vi "motorcontrol.vi"(0 "Ring":u16(ring) items=["Horizontal", "Vertical"], 1 "Direction":bool=TRUE, 2 "Frequency":dbl, 3 "# of steps":i32=1000, 4 "error in":errorcluster) -> (5 "error out":errorcluster)   [LabVIEW 2018]
uses:
  <vilib>/DAQmx/write.llb/DAQmx Write (Digital Bool 1Line 1Point).vi
  <vilib>/DAQmx/create/channels.llb/DAQmx Create Channel (DO-Digital Output).vi
  <vilib>/DAQmx/miscellaneous.llb/DAQmx Fill In Error Info.vi
  <vilib>/DAQmx/create/channels.llb/DAQmx Create Channel (CO-Pulse Generation-Frequency).vi
  <vilib>/DAQmx/configure/timing.llb/DAQmx Timing (Implicit).vi
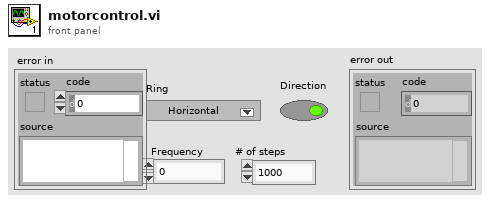
[diagram p1: front panel]
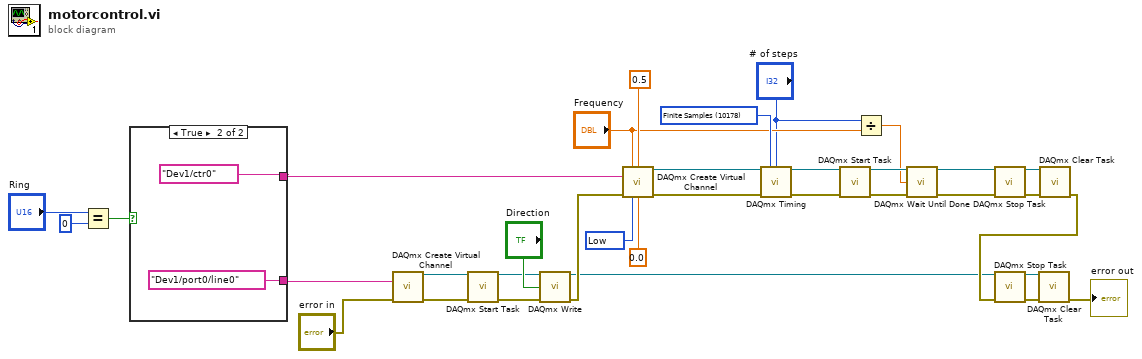
[diagram p0: block diagram]
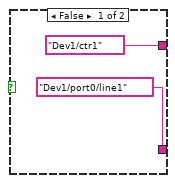
[diagram p2: hidden frame]
diagram:
  w26 = 10214 items=["High"=10192, "Low"=10214] ("idle state")
  w34 = 10178 items=["Finite Samples"=10178, "Continuous Samples"=10123, "Hardware Timed Single Point"=12522] ("sample mode")
  n1 = Equal?(x="Ring", y=u16 0) -> (x = y?=w31:bool)
  n2 = case shown="True" w31 {
    tunnel: [tag "Dev1/ctr1" ("counter") tag "Dev1/ctr0" ("counter")] -> w24
    tunnel: [tag "Dev1/port0/line1" ("lines") tag "Dev1/port0/line0" ("lines")] -> w23
    frame False {
    }
    frame True {
    }
  }
  n3 = call-poly <vilib>:"DAQmx Create Virtual Channel.vi"("lines"=w23, "error in"="error in") -> ("task out"=w22:refnum<k21>, "error out"=w21:errorcluster)  [unwired: 12 in]
  n4 = call <vilib>:"DAQmx Start Task.vi"("task/channels in"=w22, "error in"=w21) -> ("task out"=w19:refnum<k21>, "error out"=w18:errorcluster)  [unwired: 12 in]
  n5 = call-poly <vilib>:"DAQmx Write.vi"("task/channels in"=w19, "data"="Direction", "error in"=w18) -> ("task out"=w3:refnum<k21>, "error out"=w10:errorcluster)  [unwired: 10 in, 1 out]
  n6 = call-poly <vilib>:"DAQmx Create Virtual Channel.vi"("frequency"="Frequency", "duty cycle"=0.5, "counter"=w24, "error in"=w10, "idle state"=w26, "initial delay"=0.0) -> ("task out"=w9:refnum<k21>, "error out"=w8:errorcluster)  [unwired: 8 in]
  n7 = call-poly <vilib>:"DAQmx Timing.vi"("task/channels in"=w9, "sample mode"=w34, "samples per channel"="# of steps", "error in"=w8) -> ("task out"=w29:refnum<k21>, "error out"=w28:errorcluster)  [unwired: 10 in]
  n8 = call <vilib>:"DAQmx Start Task.vi"("task/channels in"=w29, "error in"=w28) -> ("task out"=w7:refnum<k21>, "error out"=w25:errorcluster)  [unwired: 12 in]
  n9 = Divide(x="# of steps", y="Frequency") -> (x/y=w4:dbl)
  n10 = call <vilib>:"DAQmx Wait Until Done.vi"("task/channels in"=w7, "timeout (sec)"=w4, "error in"=w25) -> ("task out"=w15:refnum<k21>, "error out"=w13:errorcluster)  [unwired: 11 in]
  n11 = call <vilib>:"DAQmx Stop Task.vi"("task/channels in"=w15, "error in"=w13) -> ("task out"=w27:refnum<k21>, "error out"=w12:errorcluster)  [unwired: 12 in]
  n12 = call <vilib>:"DAQmx Clear Task.vi"("task in"=w27, "error in"=w12) -> ("error out"=w11:errorcluster)  [unwired: 13 in]
  n13 = call <vilib>:"DAQmx Stop Task.vi"("task/channels in"=w3, "error in"=w11) -> ("task out"=w17:refnum<k21>, "error out"=w16:errorcluster)  [unwired: 12 in]
  n14 = call <vilib>:"DAQmx Clear Task.vi"("task in"=w17, "error in"=w16) -> ("error out"=→"error out":errorcluster)  [unwired: 13 in]
